vi "Change_Duty_Cycle_Write_VI.vi"() -> ()   [LabVIEW 2020]
uses:
  <vilib>/Utility/error.llb/DialogType.ctl
  <vilib>/DAQmx/write.llb/DAQmx Write (Counter Frequency 1Chan 1Samp).vi
  <vilib>/DAQmx/create/channels.llb/DAQmx Create Channel (CO-Pulse Generation-Frequency).vi
  <vilib>/DAQmx/configure/timing.llb/DAQmx Timing (Implicit).vi
  <vilib>/DAQmx/miscellaneous.llb/DAQmx Fill In Error Info.vi
  <resource>/objmgr/daqmx.rc
panel:
  out "duty cycle":dbl
  out "DutyCycleValue":dbl
  in  "stop":bool
  in  "pulse width":dbl=1200.0
  in  "frequency":dbl=100.0 format="%.6f"
  in  "counter":tag="Dev2/ctr1"
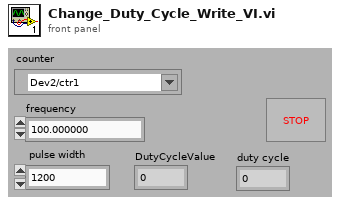
[diagram p1: front panel]
types:
  T1 = typedef "DialogType.ctl" = u16
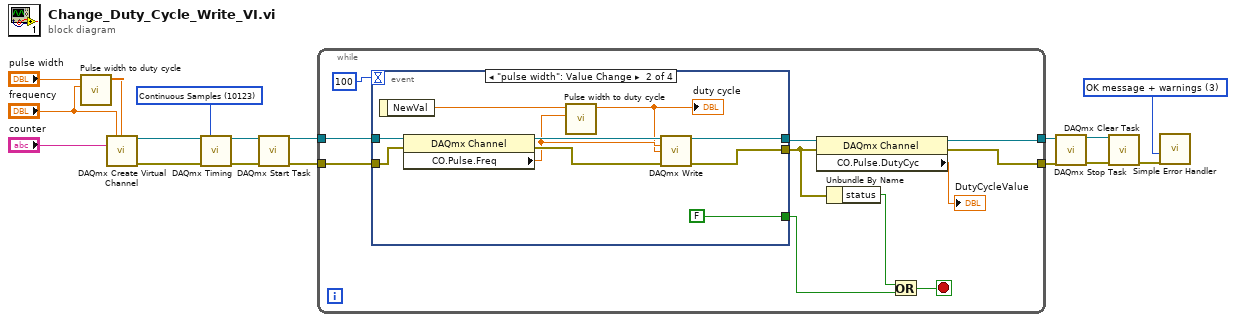
[diagram p0: block diagram]
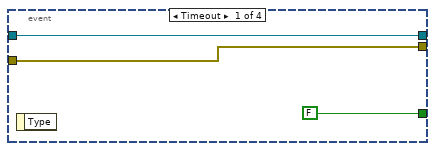
[diagram p2: hidden frame]
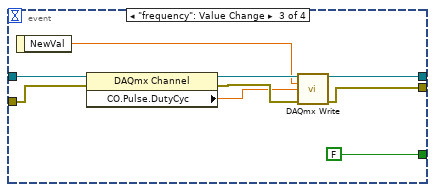
[diagram p3: hidden frame]
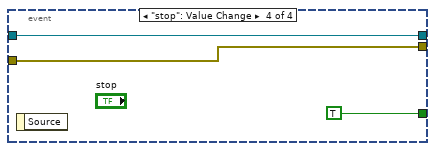
[diagram p4: hidden frame]
diagram:
  w4 = T1 3 items=["no dialog", "OK message", "continue or stop message", "OK message + warnings", "continue/stop + warnings"] ("type of dialog (OK msg:1)")
  w10 = 10123 items=["Finite Samples"=10178, "Continuous Samples"=10123, "Hardware Timed Single Point"=12522] ("sample mode")
  n1 = call "Pulse width to duty cycle.vi"("frequency"="frequency", "pulse width (us)"="pulse width") -> ("duty cycle"=w2:dbl)  [unwired: 8 in, 1 out]
  n2 = call-poly <vilib>:"DAQmx Create Virtual Channel.vi"("frequency"="frequency", "duty cycle"=w2, "counter"="counter") -> ("task out"=w17:refnum<k21>, "error out"=w16:errorcluster)  [unwired: 11 in]
  n3 = call-poly <vilib>:"DAQmx Timing.vi"("task/channels in"=w17, "sample mode"=w10, "error in"=w16) -> ("task out"=w15:refnum<k21>, "error out"=w14:errorcluster)  [unwired: 11 in]
  n4 = call <vilib>:"DAQmx Start Task.vi"("task/channels in"=w15, "error in"=w14) -> ("task out"=w13:refnum<k21>, "error out"=w12:errorcluster)  [unwired: 12 in]
  n5 = while {
    tunnel: w13 -> [w25]
    tunnel: w12 -> [w24]
    tunnel: [w19] -> w8
    tunnel: [w22] -> w9
    stop <- w27 stop-if-true
    n6 = event shown="[1] \"pulse width\": Value Change" {
      selector: _ -> [_ _ _ _]
      dyn-events: _ -> [_ _ _ _]
      timeout: 100 -> [_ _ _ _]
      tunnel: w25 -> [w30 w40 w49 w53]
      tunnel: w24 -> [w29 w39 w48 w52]
      tunnel: [w30 w36 w45 w53] -> w21
      tunnel: [w29 w35 w44 w52] -> w20
      tunnel: [FALSE FALSE FALSE TRUE] -> w23
      event Timeout {
        n7 = event-data() -> ()  [unwired: 1 in, 1 out]
      }
      event "pulse width": Value Change {
        n8 = event-data() -> ("NewVal"=w34:dbl)  [unwired: 1 in]
        n9 = property class="DAQmx Channel"(reference=w40, error in=w39) -> (reference out=w38:refnum<k21>, error out=w37:errorcluster, "CO.Pulse.Freq"=w33:dbl)
        n10 = call "Pulse width to duty cycle.vi"("frequency"=w33, "pulse width (us)"=w34) -> ("duty cycle"=w32:dbl)  [unwired: 8 in, 1 out]
        "duty cycle" <- w32
        n11 = call-poly <vilib>:"DAQmx Write.vi"("task/channels in"=w38, "frequency"=w33, "duty cycle"=w32, "error in"=w37) -> ("task out"=w36:refnum<k21>, "error out"=w35:errorcluster)  [unwired: 9 in, 1 out]
      }
      event "frequency": Value Change {
        n12 = event-data() -> ("NewVal"=w42:dbl)  [unwired: 1 in]
        n13 = property class="DAQmx Channel"(reference=w49, error in=w48) -> (reference out=w47:refnum<k21>, error out=w46:errorcluster, "CO.Pulse.DutyCyc"=w43:dbl)
        n14 = call-poly <vilib>:"DAQmx Write.vi"("task/channels in"=w47, "frequency"=w42, "duty cycle"=w43, "error in"=w46) -> ("task out"=w45:refnum<k21>, "error out"=w44:errorcluster)  [unwired: 9 in, 1 out]
      }
      event "stop": Value Change {
        n15 = event-data() -> ()  [unwired: 1 in, 1 out]
      }
    }
    n16 = property class="DAQmx Channel"(reference=w21, error in=w20) -> (reference out=w22:refnum<k21>, error out=w19:errorcluster, "CO.Pulse.DutyCyc"=→"DutyCycleValue":dbl)
    n17 = Unbundle By Name(w20) -> ("status"=w28:bool)
    n18 = Or(x=w28, y=w23) -> (x .or. y?=w27:bool)
  }
  n19 = call <vilib>:"DAQmx Stop Task.vi"("task/channels in"=w9, "error in"=w8) -> ("task out"=w7:refnum<k21>, "error out"=w6:errorcluster)  [unwired: 12 in]
  n20 = call <vilib>:"DAQmx Clear Task.vi"("task in"=w7, "error in"=w6) -> ("error out"=w5:errorcluster)  [unwired: 13 in]
  n21 = call <vilib>:"Simple Error Handler.vi"("type of dialog (OK msg:1)"=w4, "error in (no error)"=w5) -> ()  [unwired: 3 in, 5 out]
